vi "Create FileIO Process.vi"() -> (3 "File Logging Process UE Refnum":T1)   [LabVIEW 2011]
doc: "Creates the File Logging Process UE Refum.File Logging user event and File Logging Process UE Refnum.Error user event."
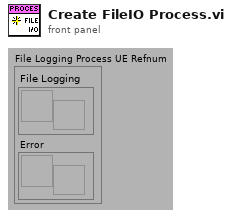
[diagram p1: front panel]
types:
  T1 = cluster{"File Logging":refnum<user-event>, "Error":refnum<user-event>}
  T2 = cluster{"Time of Step":timestamp, "# Files":i32, "Filename":path}
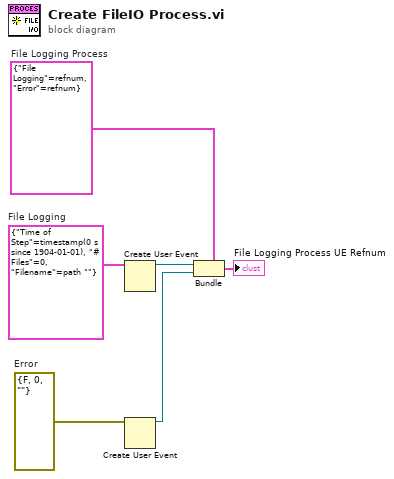
[diagram p0: block diagram]
diagram:
  w4 = T1 {"File Logging"=refnum, "Error"=refnum}  # File Logging Process
  w5 = errorcluster {"status"=FALSE, "code"=0, "source"=""}  # Error
  w6 = T2 {"Time of Step"=timestamp(0 s since 1904-01-01), "# Files"=0, "Filename"=path ""}  # File Logging
  n1 = Create User Event(user event datatype=w6) -> (user event=w3:refnum<user-event>)  [unwired: 1 in, 1 out]
  n2 = Create User Event(user event datatype=w5) -> (user event=w2:refnum<user-event>)  [unwired: 1 in, 1 out]
  n3 = Bundle(cluster=w4, "File Logging"=w3, "Error"=w2) -> (→"File Logging Process UE Refnum":T1)
